vi "!Test-Sgraph-system.vi"() -> ()   [LabVIEW 2020]
uses:
  <vilib>/Platform/TimedLoop/XDataNode/timing_clust.ctl
  <vilib>/Platform/TimedLoop/XDataNode/nitl_modes.ctl
  <vilib>/Platform/TimedLoop/XDataNode/wakeup.ctl
  Common/controls/Global-services.vi
  <vilib>/platform/TimedLoop/XDataNode/XDataNode.xnode
  <vilib>/Platform/TimedLoop/XDataNode/XDNodeRunTimeDep.lvlib
  Gserver/Gserver.lvclass
  HISW/HISW.lvclass
panel:
  in  "DBAL":bool
  in  "M Map":bool caption="Memory Map"
  out "HISW-queue":i32
  in  "OpenGraph":bool caption="Graph"
  out "HMI-error":bool
  out "Numeric":i32
  in  "Gserver":bool
  in  "FAMM":bool
  in  "HISW":bool
  in  "Stop DAQ":bool
  out "DAQ":picture
  in  "DAQ":bool
  # "Test Sgraph data historian test utility"
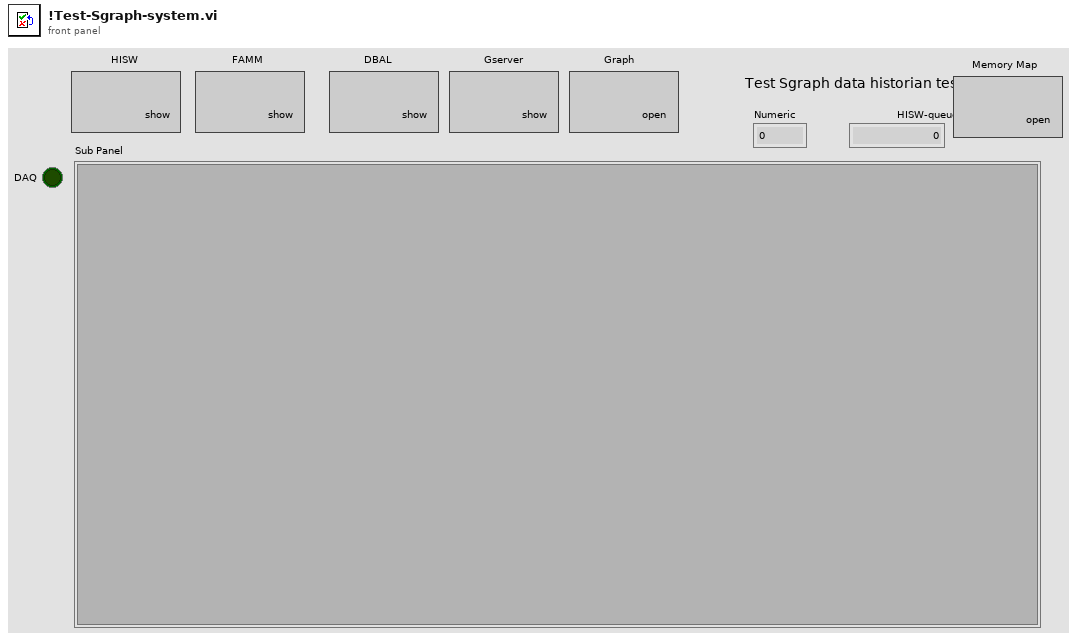
[diagram p1: front panel]
types:
  T1 = typedef "XDNodeRunTimeDep.lvlib/timing_clust.ctl" = cluster{"Expected End [f-1]":u64, "Actual End [f-1]":u64, "Finished Late? [f-1]":bool, "Expected End [i-1]":u64, "Actual End [i-1]":u64, "Finished Late? [i-1]":bool, "Expected Start [i]":u64, "Actual Start [i]":u64, "Expected Start [f]":u64, "Actual Start [f]":u64, "Source Name":string, "Structure Name":string, "Period":i64, "Deadline":i64, "Offset":i64, "Start":i64, "Priority":i32, "Timeout":i32, "Mode":T2, "Wakeup Reason":T3, "Error":errorcluster, "Source Type":string, "Secondary Source Type":string, "Global End Time":u64, "Global Start Time":u64, "Frame Duration":u64, "Iteration Duration":u64, "Assigned CPU":i32, "I/O Scan Engine Mode":u32}
  T2 = typedef "XDNodeRunTimeDep.lvlib/nitl_modes.ctl" = enum32{"No Change", "Process missed periods, maintain original phase", "Discard missed periods, maintain original phase", "Process missed periods, ignore original phase", "Discard missed periods, ignore original phase"}
  T3 = typedef "XDNodeRunTimeDep.lvlib/wakeup.ctl" = enum32{"Normal", "Aborted", "Asynchronous wakeup", "Timing source error", "Timed loop error", "Timeout"}
  T4 = typedef "typedef_PAQsample.ctl" = cluster{"Time Stamp":timestamp, "TAGs":string[], "status":u32[], "data":dbl[], "Source":string}
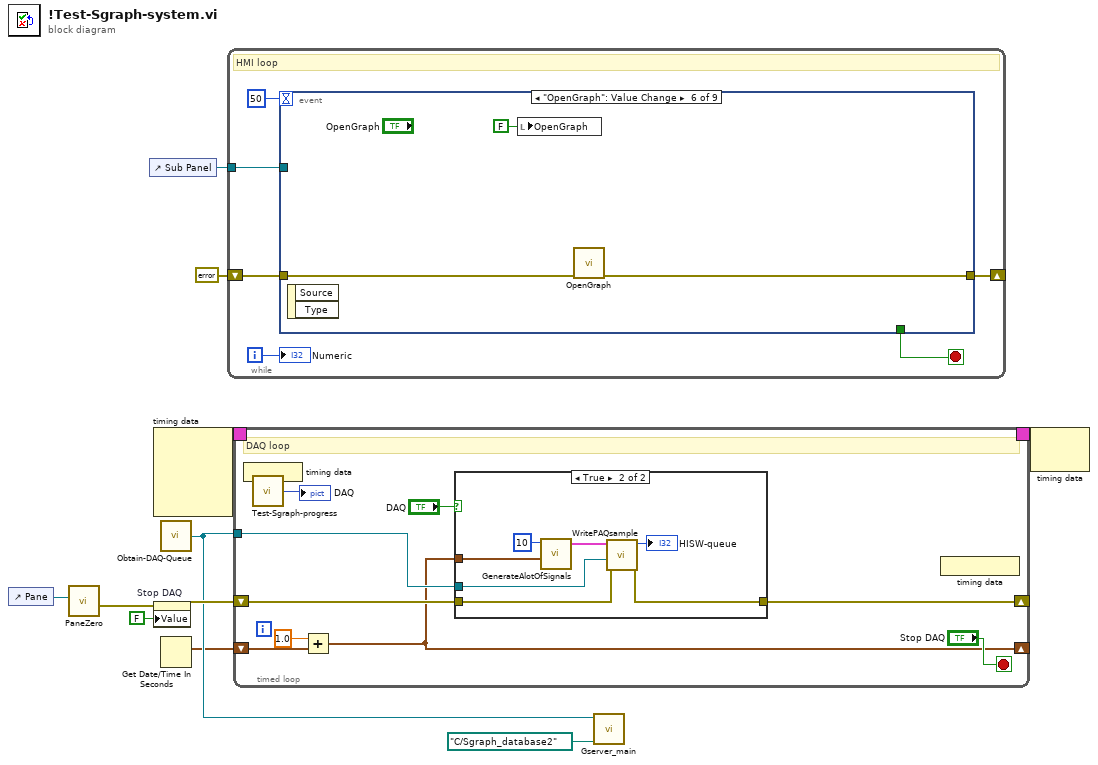
[diagram p0: block diagram]
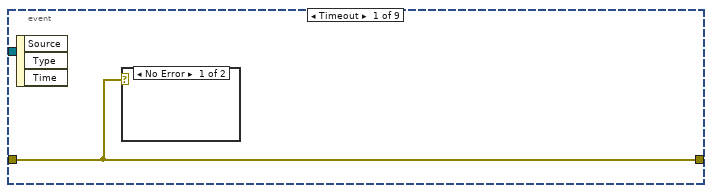
[diagram p3: hidden frame]
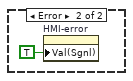
[diagram p4: hidden frame]
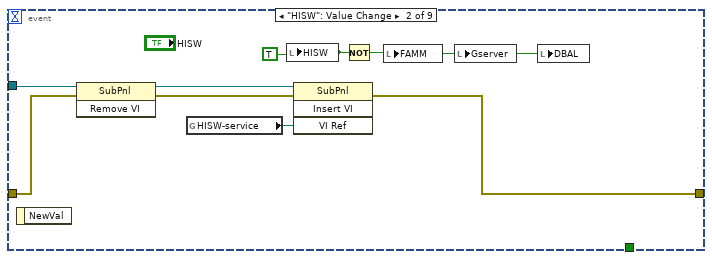
[diagram p5: hidden frame]
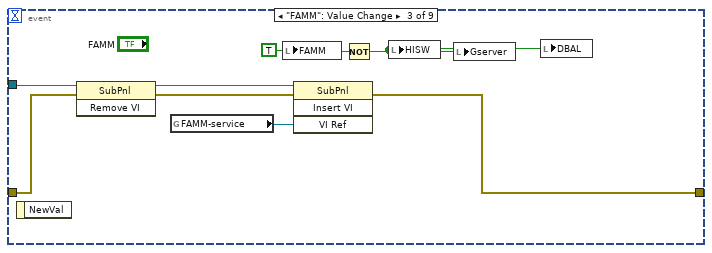
[diagram p6: hidden frame]
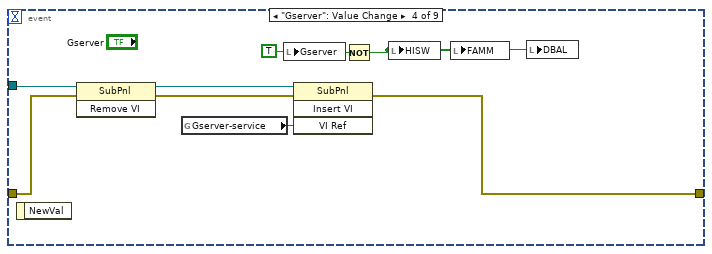
[diagram p7: hidden frame]
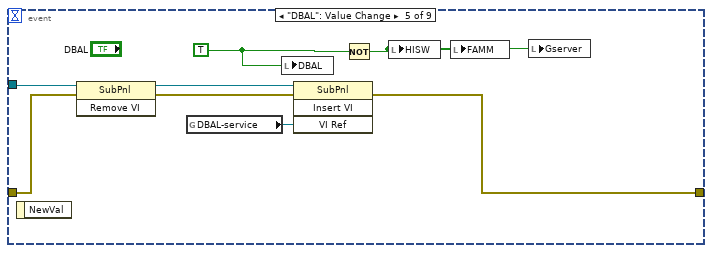
[diagram p8: hidden frame]
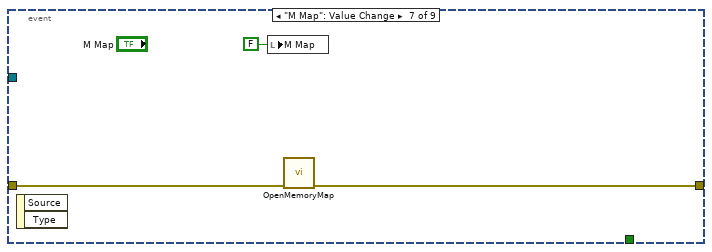
[diagram p9: hidden frame]
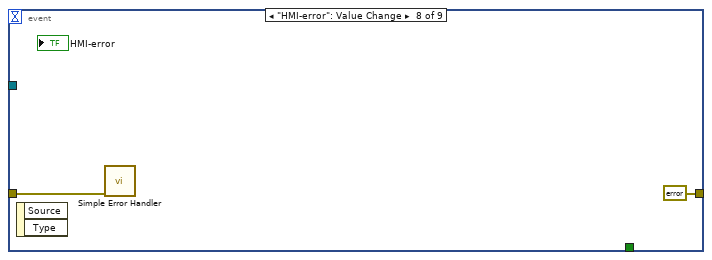
[diagram p10: hidden frame]
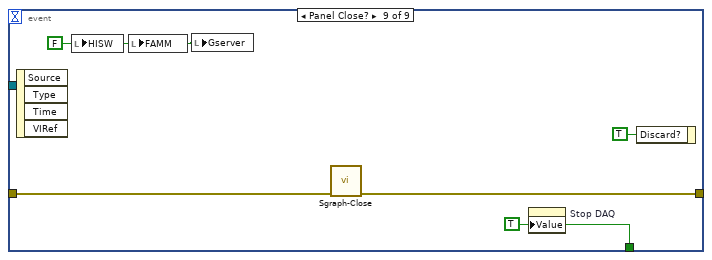
[diagram p11: hidden frame]
diagram:
  n1 = control-ref of="Pane"() -> (w4:refnum<vi>)
  n2 = call "PaneZero.vi"("Pane"=w4) -> ("error out"=w5:errorcluster)  [unwired: 10 in]
  n3 = control-ref of="Sub Panel"() -> (w7:refnum<vi>)
  n4 = node-c288() -> (w11:T1)  [unwired: 4 in]
  n5 = property on="Stop DAQ" class="Bool (strict)"(error in=w5, "Value"=FALSE ("Stop DAQ")) -> (error out=w8:errorcluster)  [unwired: 1 in, 1 out]
  n6 = call "Obtain-DAQ-Queue.vi"() -> ("DAQ-Queue"=w3:refnum<queue>)  [unwired: 7 in]
  n7 = Get Date/Time In Seconds() -> (seconds since 1Jan1904=w2:timestamp)
  n8 = while {
    tunnel: w7 -> [w16]
    shift-right: [w15] -> _
    shift-left: errorcluster {"status"=FALSE, "code"=0, "source"=""} ("error out") -> [w14]
    i -> [w12]
    stop <- w13 stop-if-true
    # "HMI loop"
    n9 = event shown="[5] \"OpenGraph\": Value Change" {
      selector: _ -> [_ _ _ _ _ _ _ _ _]
      dyn-events: _ -> [_ _ _ _ _ _ _ _ _]
      timeout: 50 -> [_ _ _ _ _ _ _ _ _]
      tunnel: [_ _ _ _ _ _ _ _ w63] -> w13
      tunnel: w16 -> [_ w26 w35 w43 w51 _ _ _ _]
      tunnel: [w18 w22 w31 w39 w47 w53 w57 errorcluster {"status"=FALSE, "code"=0, "source"=""} ("error out") w61] -> w15
      tunnel: w14 -> [w18 w21 w30 w38 w46 w52 w56 w58 w62]
      event Timeout {
        n10 = event-data() -> ()  [unwired: 1 in, 3 out]
        n11 = case shown="No Error" w18 {
          frame No Error {
          }
          frame Error {
            n12 = property on="HMI-error" class="Bool (strict)"("Val(Sgnl)"=TRUE ("Value (Signaling)")) -> ()  [unwired: 2 in, 2 out]
          }
        }
      }
      event "HISW": Value Change {
        w27 = TRUE ("HISW")
        n13 = event-data() -> ()  [unwired: 1 in, 1 out]
        n14 = invoke class="SubPnl" method="Remove VI"(reference=w26, error in=w21) -> (reference out=w25:refnum<vi>, error out=w23:errorcluster)  [unwired: 1 in, 1 out]
        n15 = global read "Global-services.vi" "HISW-service"() -> (w24:refnum<vi>)
        n16 = local write "HISW"(w27) -> ()
        n17 = invoke class="SubPnl" method="Insert VI"(reference=w25, error in=w23, "VI Ref"=w24) -> (error out=w22:errorcluster)  [unwired: 1 in, 3 out]
        n18 = Not(x=w27) -> (.not. x?=w20:bool)
        n19 = local write "FAMM"(w20) -> ()
        n20 = local write "Gserver"(w20) -> ()
        n21 = local write "DBAL"(w20) -> ()
      }
      event "FAMM": Value Change {
        w29 = TRUE ("HISW")
        n22 = event-data() -> ()  [unwired: 1 in, 1 out]
        n23 = invoke class="SubPnl" method="Remove VI"(reference=w35, error in=w30) -> (reference out=w34:refnum<vi>, error out=w32:errorcluster)  [unwired: 1 in, 1 out]
        n24 = global read "Global-services.vi" "FAMM-service"() -> (w33:refnum<vi>)
        n25 = local write "FAMM"(w29) -> ()
        n26 = invoke class="SubPnl" method="Insert VI"(reference=w34, error in=w32, "VI Ref"=w33) -> (error out=w31:errorcluster)  [unwired: 1 in, 3 out]
        n27 = Not(x=w29) -> (.not. x?=w28:bool)
        n28 = local write "HISW"(w28) -> ()
        n29 = local write "Gserver"(w28) -> ()
        n30 = local write "DBAL"(w28) -> ()
      }
      event "Gserver": Value Change {
        w37 = TRUE ("HISW")
        n31 = event-data() -> ()  [unwired: 1 in, 1 out]
        n32 = invoke class="SubPnl" method="Remove VI"(reference=w43, error in=w38) -> (reference out=w42:refnum<vi>, error out=w40:errorcluster)  [unwired: 1 in, 1 out]
        n33 = global read "Global-services.vi" "Gserver-service"() -> (w41:refnum<vi>)
        n34 = local write "Gserver"(w37) -> ()
        n35 = invoke class="SubPnl" method="Insert VI"(reference=w42, error in=w40, "VI Ref"=w41) -> (error out=w39:errorcluster)  [unwired: 1 in, 3 out]
        n36 = Not(x=w37) -> (.not. x?=w36:bool)
        n37 = local write "HISW"(w36) -> ()
        n38 = local write "FAMM"(w36) -> ()
        n39 = local write "DBAL"(w36) -> ()
      }
      event "DBAL": Value Change {
        w45 = TRUE ("HISW")
        n40 = event-data() -> ()  [unwired: 1 in, 1 out]
        n41 = invoke class="SubPnl" method="Remove VI"(reference=w51, error in=w46) -> (reference out=w50:refnum<vi>, error out=w48:errorcluster)  [unwired: 1 in, 1 out]
        n42 = global read "Global-services.vi" "DBAL-service"() -> (w49:refnum<vi>)
        n43 = local write "DBAL"(w45) -> ()
        n44 = invoke class="SubPnl" method="Insert VI"(reference=w50, error in=w48, "VI Ref"=w49) -> (error out=w47:errorcluster)  [unwired: 1 in, 3 out]
        n45 = Not(x=w45) -> (.not. x?=w44:bool)
        n46 = local write "HISW"(w44) -> ()
        n47 = local write "FAMM"(w44) -> ()
        n48 = local write "Gserver"(w44) -> ()
      }
      event "OpenGraph": Value Change {
        n49 = event-data() -> ()  [unwired: 1 in, 2 out]
        n50 = local write "OpenGraph"(FALSE ("OpenGraph")) -> ()
        n51 = call "OpenGraph.vi"("error in (no error)"=w52) -> ("Error out"=w53:errorcluster)  [unwired: 10 in]
      }
      event "M Map": Value Change {
        n52 = event-data() -> ()  [unwired: 1 in, 2 out]
        n53 = local write "M Map"(FALSE ("M Map")) -> ()
        n54 = call "OpenMemoryMap.vi"("error in (no error)"=w56) -> ("Error out"=w57:errorcluster)  [unwired: 10 in]
      }
      event "HMI-error": Value Change {
        n55 = event-data() -> ()  [unwired: 1 in, 2 out]
        n56 = call <vilib>:"Simple Error Handler.vi"("error in (no error)"=w58) -> ()  [unwired: 4 in, 5 out]
      }
      event Panel Close? {
        w60 = FALSE ("HISW")
        w63 = TRUE ("Stop DAQ")
        n57 = event-data() -> ()  [unwired: 1 in, 4 out]
        n58 = local write "HISW"(w60) -> ()
        n59 = local write "FAMM"(w60) -> ()
        n60 = local write "Gserver"(w60) -> ()
        n61 = call "Sgraph-Close.vi"("error in (no error)"=w62) -> ("error out"=w61:errorcluster)  [unwired: 10 in]
        n62 = property on="Stop DAQ" class="Bool (strict)"("Value"=w63) -> ()  [unwired: 2 in, 2 out]
        n63 = event-data("Discard?"=TRUE) -> ()  [unwired: 1 in, 1 out]
      }
    }
    "Numeric" <- w12
  }
  n64 = timed-loop {
    timing: w11 -> [_]
    timing-out: [_] -> w10
    shift-right: [w69] -> _
    shift-left: w8 -> [w70]
    tunnel: w3 -> [w68]
    shift-right: [w65] -> _
    shift-left: w2 -> [w67]
    stop <- "Stop DAQ" stop-if-true
    # "DAQ loop"
    n65 = node-c288() -> ()  [unwired: 1 in]
    n66 = call "Test-Sgraph-progress.vi"() -> ("37x37"=→"DAQ":picture)  [unwired: 7 in]
    n67 = Add(x=1.0, y=w67) -> (x+y=w65:timestamp)
    n68 = case shown="True" "DAQ" {
      tunnel: w70 -> [w74 w79]
      tunnel: [w74 w78] -> w69
      tunnel: w68 -> [_ w77]
      tunnel: w65 -> [_ w75]
      frame False {
      }
      frame True {
        n69 = call "GenerateAlotOfSignals.vi"("Time"=w75, "Channels"=10) -> ("DAQ"=w80:T4)  [unwired: 9 in]
        n70 = call "WritePAQsample.vi"("error in (no error)"=w79, "DAQ-Queue"=w77, "PAQ IN"=w80) -> ("error out"=w78:errorcluster, "# elements in queue"=→"HISW-queue":i32)  [unwired: 7 in]
      }
    }
    n71 = node-c288() -> ()  [unwired: 1 out]
  }
  n72 = call "Gserver_main.vi"("Database location"=path "C:/Sgraph_database2", "DAQ-Queue"=w3) -> ()  [unwired: 10 in]
  n73 = node-c288(w10) -> ()  [unwired: 1 out]
